vi "MaxFound.vi"(11 "Input Y Values":dbl[](array[numeric])) -> (2 "Max?":bool, 3 "Output Y Values":dbl[](array[numeric]))   [LabVIEW 2014]
panel:
  # "Peak Finding VI"
  # "Inputs"
  # "Outputs"
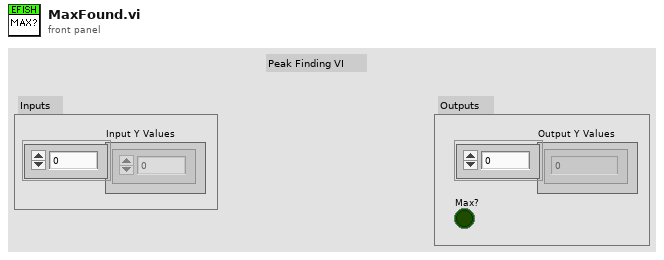
[diagram p1: front panel]
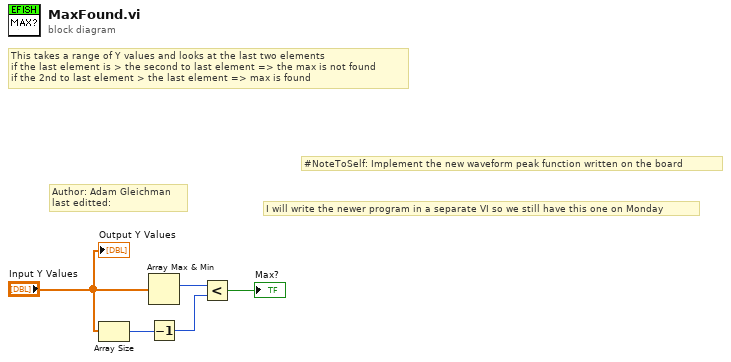
[diagram p0: block diagram]
diagram:
  # "I will write the newer program in a separate VI so we still have this one on Monday"
  # "#NoteToSelf: Implement the new waveform peak function written on the board"
  # "Author: Adam Gleichman\nlast editted:"
  # "This takes a range of Y values and looks at the last two elements\nif the last element is > the second to last element => the max is not found\nif the 2nd to last element > the last element => max is found"
  n1 = Array Size(array="Input Y Values") -> (size(s)=w4:i32)
  n2 = Array Max & Min(array="Input Y Values") -> (max index (indices)=w1:i32)  [unwired: 3 out]
  n3 = Decrement(x=w4) -> (x-1=w3:i32)
  n4 = Less?(x=w1, y=w3) -> (x < y?=→"Max?":bool)
  "Output Y Values" <- "Input Y Values"
